vi "RootBLE.vi"() -> ()   [LabVIEW 2016]
uses:
  VIs/uPythonX/uPythonX.xctl
panel:
  in  "Trinket":T1(xcontrol)={"Port"="Spike - ASRL73::INSTR", "All Code"=""}
  in  "BLE - Root":T1(xcontrol)={"Port"="Spike - ASRL73::INSTR", "All Code"="import hub,utime\nroot_identifier_uuid = '48c5d828-ac2a-442d-97a3-0c9822b04979'\ndrive_forward = [0x01, 0x04, 0x00, 0x00, 0x00, 0x00, 0x64, 0x00, 0x00, 0x00, 0x64, 0x00, 0x00, 0x00, 0x00, 0x00, 0x00, 0x00, 0x00, 0xD1]\n\nhub.ble.rssi(-70)\nhub.ble.scan(1)\nutime.sleep(1)\ndevices = hub.ble.scan_result()\n\n# foo = [x for x in fred if x['service_id'] == root_identifier_uuid.upper()]\n\ndef connect_callback(a):\n     print('Connection complete: {0}'.format(a))\n\ndesired = -1\ncounter = 0\nfor device in devices:\n     if device['service_id'] == root_identifier_uuid.upper():\n          desired = counter\n          print('found '+ str(desired))\n          print (device)\n     counter += 1\n   \nhub.ble.callback(connect_callback)\nroot = hub.ble.connect(desired)\n\n'''\n     root.send(drive_forward)\n     root.disconnect()\n'''"}
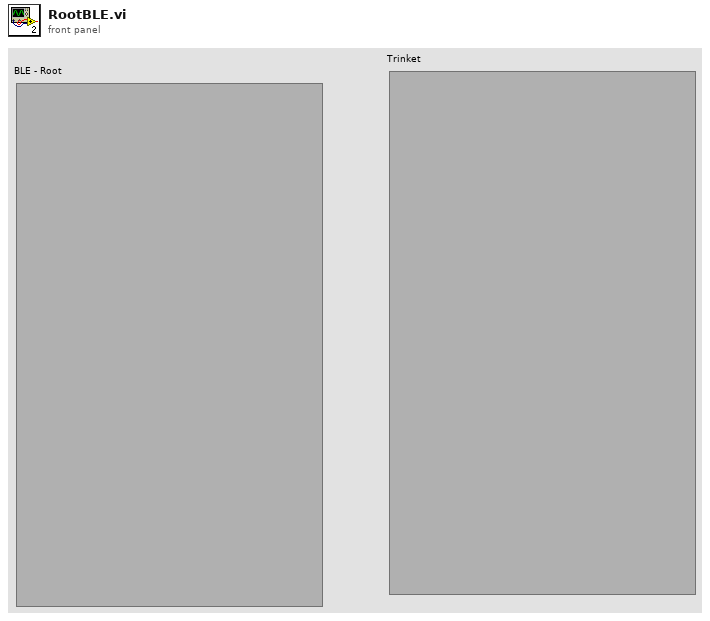
[diagram p1: front panel]
types:
  T1 = cluster{"Port":refnum<visa-resource-name>, "All Code":string}
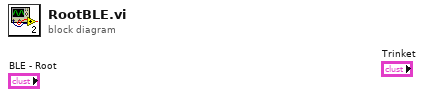
[diagram p0: block diagram]
diagram:
